vi "DHE_FormatID.vi"(8 "id counter in":u32, 9 "UT in":string, 10 "IDbase in":string) -> (2 "expID out":string)   [LabVIEW 2016]
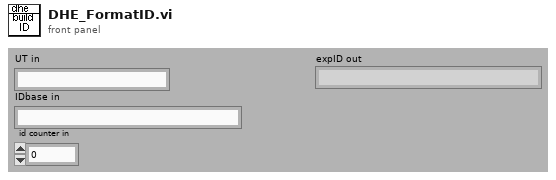
[diagram p1: front panel]
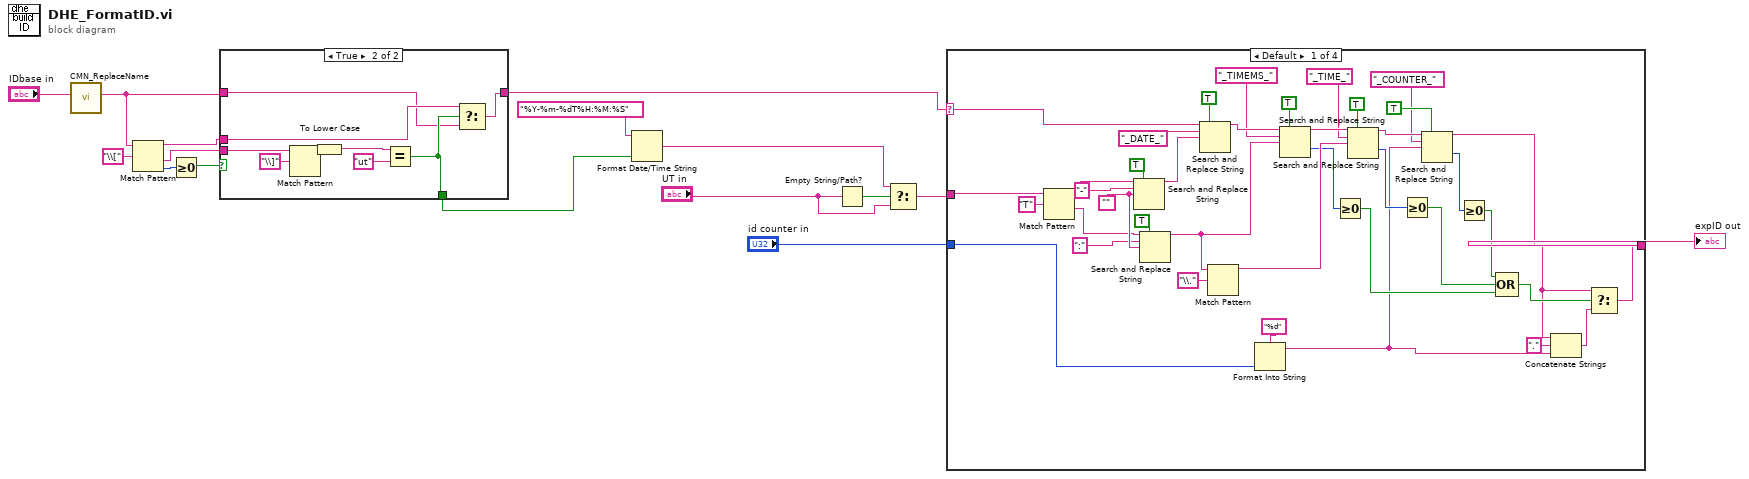
[diagram p0: block diagram]
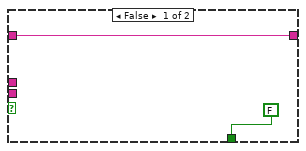
[diagram p2: hidden frame]
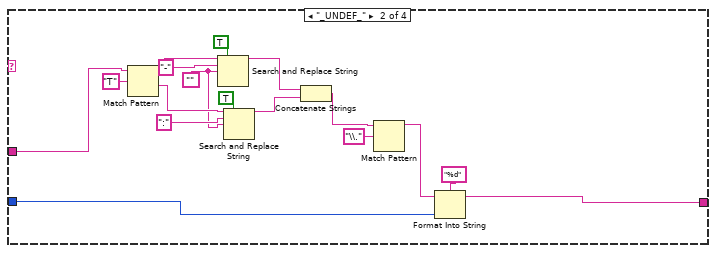
[diagram p3: hidden frame]
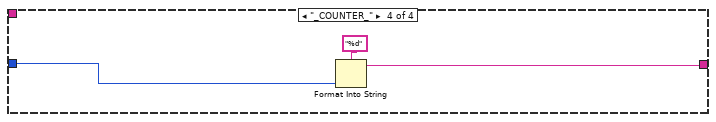
[diagram p5: hidden frame]
diagram:
  n1 = call "CMN_ReplaceName.vi"("name in"="IDbase in") -> ("name out"=w5:string)  [unwired: 1 in, 9 out]
  n2 = Match Pattern(string=w5, regular expression="\\[") -> (before substring=w3:string, after substring=w2:string, offset past match=w7:i32)  [unwired: 2 out]
  n3 = Greater Or Equal To 0?(x=w7) -> (x >= 0?=w6:bool)
  n4 = case shown="True" w6 {
    tunnel: w5 -> [w18 w19]
    tunnel: [w18 w20] -> w4
    tunnel: w3 -> [_ w21]
    tunnel: w2 -> [_ w26]
    tunnel: [FALSE w22] -> w1
    frame False {
    }
    frame True {
      n5 = Match Pattern(string=w26, regular expression="\\]") -> (before substring=w24:string)  [unwired: 4 out]
      n6 = To Lower Case(string=w24) -> (all lower case string=w23:string)
      n7 = Equal?(x=w23, y="ut") -> (x = y?=w22:bool)
      n8 = Select(t=w21, s=w22, f=w19) -> (s? t:f=w20:string)
    }
  }
  n9 = Format Date/Time String(time format string (%c)="%Y-%m-%dT%H:%M:%S", UTC format=w1) -> (date/time string=w12:string)  [unwired: 1 out]
  n10 = Empty String/Path?(string/path="UT in") -> (empty?=w13:bool)
  n11 = Select(t=w12, s=w13, f="UT in") -> (s? t:f=w10:string)
  n12 = case shown="Default" w4 {
    selector: w4 -> [w66 _ _ _]
    tunnel: w10 -> [w63 w70 w84 _]
    tunnel: "id counter in" -> [w40 w82 _ w86]
    tunnel: [w30 w81 w84 w85] -> w15
    frame Default {
      w57 = ""
      n13 = Match Pattern(string=w63, regular expression="T") -> (before substring=w61:string, after substring=w55:string)  [unwired: 3 out]
      n14 = Search and Replace String(replace all?=TRUE ("replace all? (F)"), input string=w61, search string="-", replace string=w57) -> (result string=w54:string)  [unwired: 1 in, 6 out]
      n15 = Search and Replace String(replace all?=TRUE ("replace all? (F)"), input string=w55, search string=":", replace string=w57) -> (result string=w47:string)  [unwired: 1 in, 6 out]
      n16 = Search and Replace String(replace all?=TRUE ("replace all? (F)"), input string=w66, search string="_DATE_", replace string=w54) -> (result string=w52:string)  [unwired: 1 in, 6 out]
      n17 = Match Pattern(string=w47, regular expression="\\.") -> (before substring=w45:string)  [unwired: 4 out]
      n18 = Format Into String(format string="%d", w40) -> (resulting string=w32:string)  [unwired: 2 in, 1 out]
      n19 = Search and Replace String(replace all?=TRUE ("replace all? (F)"), input string=w52, search string="_TIMEMS_", replace string=w47) -> (result string=w49:string, offset past replacement=w39:i32)  [unwired: 1 in, 5 out]
      n20 = Greater Or Equal To 0?(x=w39) -> (x >= 0?=w34:bool)
      n21 = Search and Replace String(replace all?=TRUE ("replace all? (F)"), input string=w49, search string="_TIME_", replace string=w45) -> (result string=w44:string, offset past replacement=w38:i32)  [unwired: 1 in, 5 out]
      n22 = Greater Or Equal To 0?(x=w38) -> (x >= 0?=w35:bool)
      n23 = Search and Replace String(replace all?=TRUE ("replace all? (F)"), input string=w44, search string="_COUNTER_", replace string=w32) -> (result string=w29:string, offset past replacement=w37:i32)  [unwired: 1 in, 5 out]
      n24 = Greater Or Equal To 0?(x=w37) -> (x >= 0?=w36:bool)
      n25 = Compound Arithmetic op=OR(w36, w35, w34) -> (w33:bool)
      n26 = Concatenate Strings(w29, "." ("string"), w32) -> (w31:string)
      n27 = Select(t=w29, s=w33, f=w31) -> (s? t:f=w30:string)
    }
    frame "_UNDEF_" {
      w73 = ""
      n28 = Match Pattern(string=w70, regular expression="T") -> (before substring=w79:string, after substring=w75:string)  [unwired: 3 out]
      n29 = Search and Replace String(replace all?=TRUE ("replace all? (F)"), input string=w79, search string="-", replace string=w73) -> (result string=w72:string)  [unwired: 1 in, 6 out]
      n30 = Search and Replace String(replace all?=TRUE ("replace all? (F)"), input string=w75, search string=":", replace string=w73) -> (result string=w71:string)  [unwired: 1 in, 6 out]
      n31 = Concatenate Strings(w72, w71) -> (w68:string)
      n32 = Match Pattern(string=w68, regular expression="\\.") -> (before substring=w67:string)  [unwired: 4 out]
      n33 = Format Into String(format string="%d", initial string=w67, w82) -> (resulting string=w81:string)  [unwired: 1 in, 1 out]
    }
    frame "_UT_" {
    }
    frame "_COUNTER_" {
      n34 = Format Into String(format string="%d", w86) -> (resulting string=w85:string)  [unwired: 2 in, 1 out]
    }
  }
  "expID out" <- w15
